vi "340 set Temp(SubVI).vi"(6 "Loop (0: 1)":u16(ring) items=["1", "2"], 7 "Input (0:A)":u16(ring) items=["A", "B"], 8 "error in (no error)":errorcluster, 9 "Rate":dbl=5.0, 10 "Temperature":dbl=2.0, 11 "VISA Refnum in":refnum<visa-resource-name>="GPIB0::14::INSTR") -> (0 "error out":errorcluster, 3 "VISA resource name out":refnum<visa-resource-name>)   [LabVIEW 2019]
uses:
  lib/Lake Shore 340/Lake Shore Cryotronics 340.lvlib
panel:
  out "Sensor Data":dbl format="%.4f"
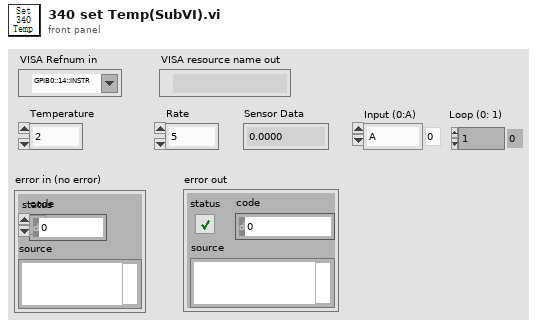
[diagram p1: front panel]
types:
  T1 = typedef "Semaphore RefNum" = refnum<k1>
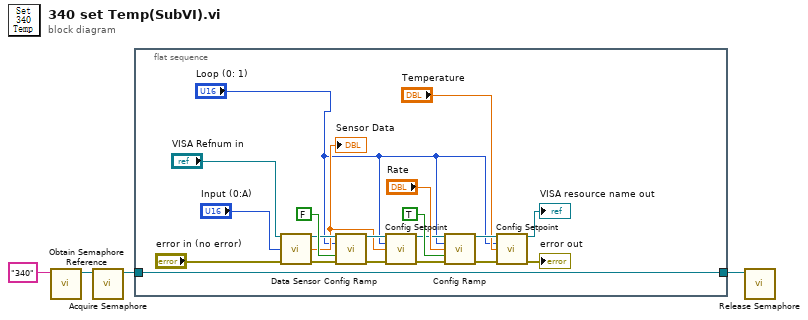
[diagram p0: block diagram]
diagram:
  n1 = call <vilib>:"Obtain Semaphore Reference.vi"("name (unnamed)"="340") -> ("semaphore"=w3:T1)  [unwired: 4 in, 2 out]
  n2 = call <vilib>:"Acquire Semaphore.vi"("semaphore"=w3) -> ("semaphore out"=w2:T1)  [unwired: 4 in, 2 out]
  n3 = flat-sequence {
    tunnel: w2 -> [w22]
    tunnel: [w22] -> w1
    frame #0 {
      n4 = call "Data Sensor.vi"("VISA resource name"="VISA Refnum in", "Input (0: A)"="Input (0:A)", "error in (no error)"="error in (no error)") -> ("VISA resource name out"=w8:refnum<visa-resource-name>, "Kelvin Reading"=w6:dbl, "error out"=w17:errorcluster)  [unwired: 8 in, 2 out]
      "Sensor Data" <- w6
      n5 = call "Config Ramp.vi"("VISA resource name"=w8, "Loop (0: 1)"="Loop (0: 1)", "Ramping On/Off (F: Ramping Off)"=FALSE ("Enable Setpoint Ramping (F: Off)"), "error in (no error)"=w17) -> ("VISA resource name out"=w12:refnum<visa-resource-name>, "error out"=w20:errorcluster)  [unwired: 10 in]
      n6 = call "Config Setpoint.vi"("VISA resource name"=w12, "Loop (0: 1)"="Loop (0: 1)", "Setpoint (0.0)"=w6, "error in (no error)"=w20) -> ("VISA resource name out"=w11:refnum<visa-resource-name>, "error out"=w19:errorcluster)  [unwired: 10 in]
      n7 = call "Config Ramp.vi"("VISA resource name"=w11, "Loop (0: 1)"="Loop (0: 1)", "Rate Value (0.1)"="Rate", "Ramping On/Off (F: Ramping Off)"=TRUE ("Enable Setpoint Ramping (F: Off)"), "error in (no error)"=w19) -> ("VISA resource name out"=w10:refnum<visa-resource-name>, "error out"=w18:errorcluster)  [unwired: 9 in]
      n8 = call "Config Setpoint.vi"("VISA resource name"=w10, "Loop (0: 1)"="Loop (0: 1)", "Setpoint (0.0)"="Temperature", "error in (no error)"=w18) -> ("VISA resource name out"=→"VISA resource name out":refnum<visa-resource-name>, "error out"=→"error out":errorcluster)  [unwired: 10 in]
    }
  }
  n9 = call <vilib>:"Release Semaphore.vi"("semaphore"=w1) -> ()  [unwired: 5 in, 2 out]
